vi "Repack Package.vi"(4 "Delete Directory to repack (TRUE)?":bool=TRUE, 6 "Overwrite Target Package File (True)?":bool=TRUE, 7 "Package File (\"\": use name of directory to repack)":path, 8 "error in (no error)":errorcluster, 11 "Directory to repack":path) -> (0 "error out":errorcluster)   [LabVIEW 2024]
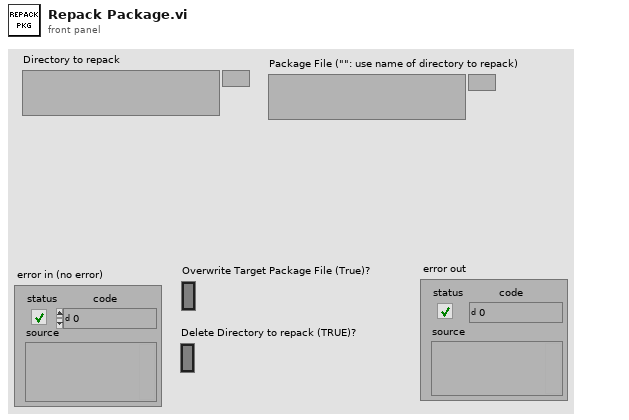
[diagram p1: front panel]
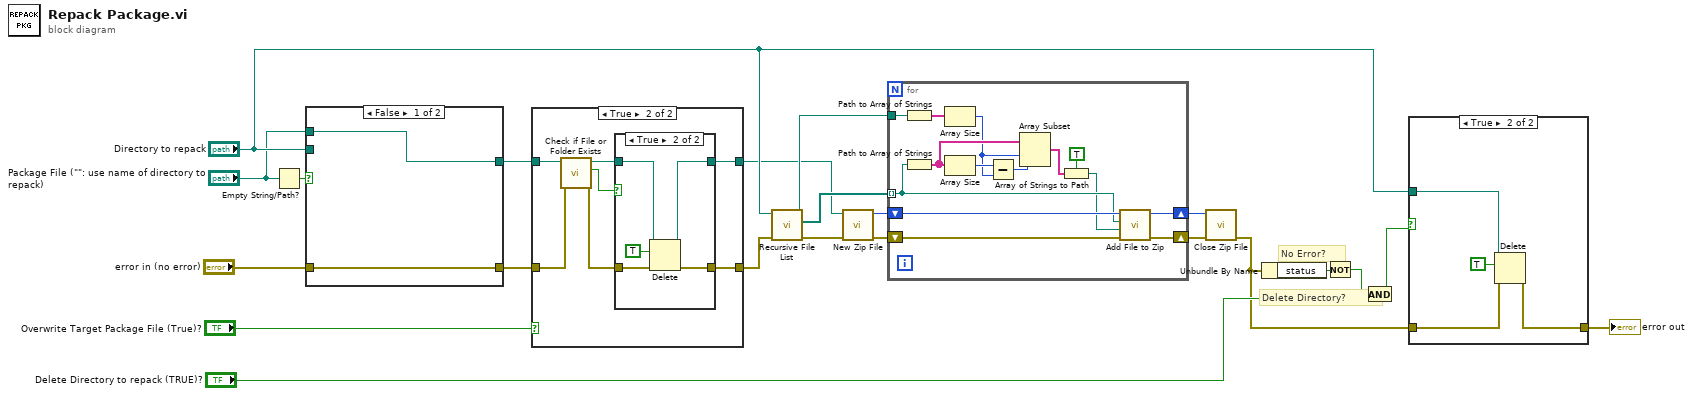
[diagram p0: block diagram]
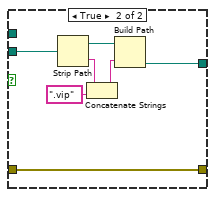
[diagram p4: hidden frame]
diagram:
  # "Delete Directory?"
  # "No Error?"
  n1 = Empty String/Path?(string/path="Package File (\"\": use name of directory to repack)") -> (empty?=w22:bool)
  n2 = case shown="False" w22 {
    tunnel: "Package File (\"\": use name of directory to repack)" -> [w23 _]
    tunnel: "error in (no error)" -> [w24 w26]
    tunnel: [w24 w26] -> w20
    tunnel: [w23 w30] -> w19
    tunnel: "Directory to repack" -> [_ w25]
    frame False {
    }
    frame True {
      n3 = Strip Path(path=w25) -> (stripped path=w31:path, name=w29:string)
      n4 = Concatenate Strings(w29, ".vip" ("string")) -> (w28:string)
      n5 = Build Path(base path=w31, name or relative path=w28) -> (appended path=w30:path)
    }
  }
  n6 = case shown="True" "Overwrite Target Package File (True)?" {
    tunnel: w20 -> [w32 w40]
    tunnel: w19 -> [w33 w39]
    tunnel: [w33 w35] -> w1
    tunnel: [w32 w34] -> w17
    frame False {
    }
    frame True {
      n7 = call <vilib>:"Check if File or Folder Exists.vi"("error in (no error)"=w40, "path"=w39) -> ("error out"=w37:errorcluster, "file or folder exists?"=w38:bool, "dup path"=w36:path)  [unwired: 7 in]
      n8 = case shown="True" w38 {
        tunnel: w37 -> [w42 w47]
        tunnel: w36 -> [w41 w45]
        tunnel: [w41 w44] -> w35
        tunnel: [w42 w43] -> w34
        frame False {
        }
        frame True {
          n9 = Delete(path (use dialog)=w45, entire hierarchy (F)=TRUE, error in=w47) -> (deleted path=w44:path, error out=w43:errorcluster)  [unwired: 2 in, 1 out]
        }
      }
    }
  }
  n10 = call <vilib>:"Recursive File List.vi"("error in (no error)"=w17, "Folder Path"="Directory to repack") -> ("error out"=w16:errorcluster, "All Files in Dir"=w15:path[], "dup Folder Path"=w10:path)  [unwired: 5 in, 2 out]
  n11 = call <vilib>:"New Zip File.vi"("error in (no error)"=w16, "target"=w1) -> ("error out"=w14:errorcluster, "zip file out"=w13:i64)  [unwired: 3 in, 1 out]
  n12 = for {
    tunnel: w15 -> [w56] mode=indexing
    shift-right: [w59] -> w12
    shift-left: w14 -> [w61]
    shift-right: [w58] -> w11
    shift-left: w13 -> [w60]
    tunnel: w10 -> [w57]
    n13 = Path to Array of Strings(0:w57) -> (2:w55:string[])  [unwired: 1 out]
    n14 = Path to Array of Strings(0:w56) -> (2:w54:string[])  [unwired: 1 out]
    n15 = Array Size(array=w55) -> (size(s)=w52:i32)
    n16 = Array Size(array=w54) -> (size(s)=w53:i32)
    n17 = Subtract(x=w53, y=w52) -> (x-y=w51:i32)
    n18 = Array Subset(array=w54, index=w52, length=w51) -> (w50:string[])
    n19 = Array of Strings to Path(0:w50, 1:TRUE ("relative")) -> (2:w48:path)
    n20 = call <vilib>:"Add File to Zip.vi"("error in (no error)"=w61, "destination path in zip"=w48, "source file path"=w56, "zip file in"=w60) -> ("error out"=w59:errorcluster, "zip file out"=w58:i64)  [unwired: 6 in]
  }
  n21 = call <vilib>:"Close Zip File.vi"("error in (no error)"=w12, "zip file in"=w11) -> ("error out"=w5:errorcluster)  [unwired: 5 in]
  n22 = Unbundle By Name(w5) -> ("status"=w9:bool)
  n23 = Not(x=w9) -> (.not. x?=w8:bool)
  n24 = And(x=w8, y="Delete Directory to repack (TRUE)?") -> (x .and. y?=w6:bool)
  n25 = case shown="True" w6 {
    tunnel: w5 -> [w62 w65]
    tunnel: "Directory to repack" -> [_ w64]
    tunnel: [w62 w63] -> w4
    frame False {
    }
    frame True {
      n26 = Delete(path (use dialog)=w64, entire hierarchy (F)=TRUE, error in=w65) -> (error out=w63:errorcluster)  [unwired: 2 in, 2 out]
    }
  }
  "error out" <- w4
